vi "Module Name--constant.vi"() -> (3 "Module Name":string)   [LabVIEW 2020, in "horiba.lvlib" / "DeviceManager.lvlib"]
doc: "Return the name of the module that owns this VI. \n_____\nBased on DQMH Project Template 7.0.0.1280."
uses:
  DeviceManager.lvlib
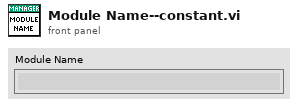
[diagram p1: front panel]
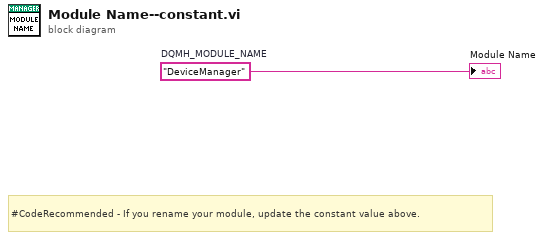
[diagram p0: block diagram]
diagram:
  w1 = "DeviceManager"  # DQMH_MODULE_NAME
  # "#CodeRecommended - If you rename your module, update the constant value above."
  "Module Name" <- w1
